vi "AlazarSetTriggerTimeOut.vi"(3 "error in (no error)":errorcluster, 4 "Timeout Ticks":u32, 5 "Handle":u32) -> (0 "error out":errorcluster, 1 "Return Code":u32, 2 "Handle":u32)   [LabVIEW 2024]
doc: "Set the time to wait for a trigger event before automatically generating a trigger event."
uses:
  ATSApi.dll
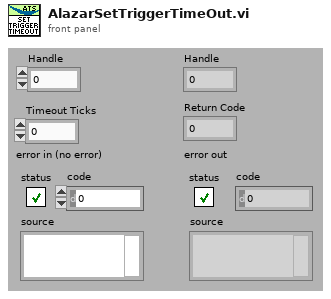
[diagram p1: front panel]
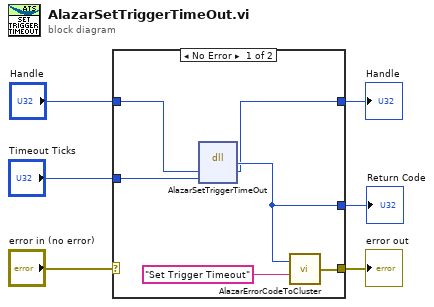
[diagram p0: block diagram]
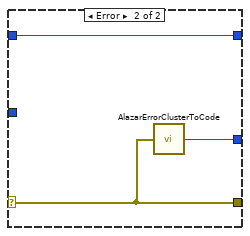
[diagram p2: hidden frame]
diagram:
  n1 = case shown="No Error" "error in (no error)" {
    selector: "error in (no error)" -> [_ w15]
    tunnel: [w9 w15] -> w5
    tunnel: [w11 w14] -> w4
    tunnel: "Handle" -> [w12 w13]
    tunnel: [w8 w13] -> w2
    tunnel: "Timeout Ticks" -> [w7 _]
    frame No Error {
      n2 = dll-call lib="ATSApi.dll" fn="AlazarSetTriggerTimeOut"("handle"=w12, "timeoutTicks"=w7) -> (w11:u32, "handle"=w8:u32)  [unwired: 4 in, 2 out]
      n3 = call "AlazarErrorCodeToCluster.vi"("Message"="Set Trigger Timeout", "Error Code"=w11) -> ("error out"=w9:errorcluster)
    }
    frame Error {
      n4 = call "AlazarErrorClusterToCode.vi"("error in (no error)"=w15) -> ("Error Code"=w14:u32)
    }
  }
  "Handle" <- w2
  "error out" <- w5
  "Return Code" <- w4
